vi "4-channel oscilloscope v1.01.vi"() -> ()   [LabVIEW 2014]
doc: "This example shows how to configure multiple channels and acquire waveforms from multiple channels."
uses:
  <vilib>/Analysis/Matrix/Datatypes/RealMatrix.ctl
  <instrlib>/Tektronix TDS 200 1000 2000 Series/Tektronix TDS 200 1000 2000 Series.lvlib
  <vilib>/Analysis/Matrix/NI_Matrix.lvlib
panel:
  out "Real Matrix":T1
  in  "Channel 4 (3: Channel 4)":u16(ring) items=["Channel 1", "Channel 2", "Channel 3", "Channel 4", "Math", "Reference A", "Reference B", "Reference C", "Reference D"]
  in  "Probe Attenuation 4 (0.1)":dbl=10.0
  in  "Vertical Coupling 4 (1: DC)":u16(ring)=1 items=["AC", "DC", "Ground"]
  in  "Channel 3 (2: Channel 3)":u16(ring) items=["Channel 1", "Channel 2", "Channel 3", "Channel 4", "Math", "Reference A", "Reference B", "Reference C", "Reference D"]
  in  "Probe Attenuation 3 (0.1)":dbl=10.0
  in  "Vertical Coupling 3 (1: DC)":u16(ring)=1 items=["AC", "DC", "Ground"]
  in  "Channel 2 (1: Channel 2)":u16(ring)=1 items=["Channel 1", "Channel 2", "Channel 3", "Channel 4", "Math", "Reference A", "Reference B", "Reference C", "Reference D"]
  in  "Channel 1 (0: Channel 1)":u16(ring) items=["Channel 1", "Channel 2", "Channel 3", "Channel 4", "Math", "Reference A", "Reference B", "Reference C", "Reference D"]
  in  "Serial Configuration":T2={"Baud Rate"=9600, "Parity"=0, "Stop Bits"=10, "Flow Control"=2} {"Flow Control" items=["None", "XON/XOFF", "RTS/CTS", "XON/XOFF & RTS/CTS", "DTR/DSR", "XON/XOFF & DTR/DSR"]; "Stop Bits" items=["1.0"=10, "1.5"=15, "2.0"=20]; "Parity" items=["None", "Odd", "Even", "Mark", "Space"]; "Baud Rate" items=["300"=300, "600"=600, "1200"=1200, "2400"=2400, "4800"=4800, "9600"=9600, "19200"=19200]}
  in  "Probe Attenuation 2 (0.1)":dbl=1.0
  in  "Vertical Coupling 2 (1: DC)":u16(ring)=1 items=["AC", "DC", "Ground"]
  in  "Probe Attenuation 1 (0.1)":dbl=10.0
  in  "Vertical Coupling 1 (1: DC)":u16(ring)=1 items=["AC", "DC", "Ground"]
  in  "Timeout (10000 ms)":u32=10000
  out "Waveform Data":waveform(dbl)[](graph)
  in  "VISA resource name":refnum<visa-resource-name>
  # "2015 NanoBEEs"
  # "Channel 3"
  # "Channel 1"
  # "Channel 2"
  # "Channel 4"
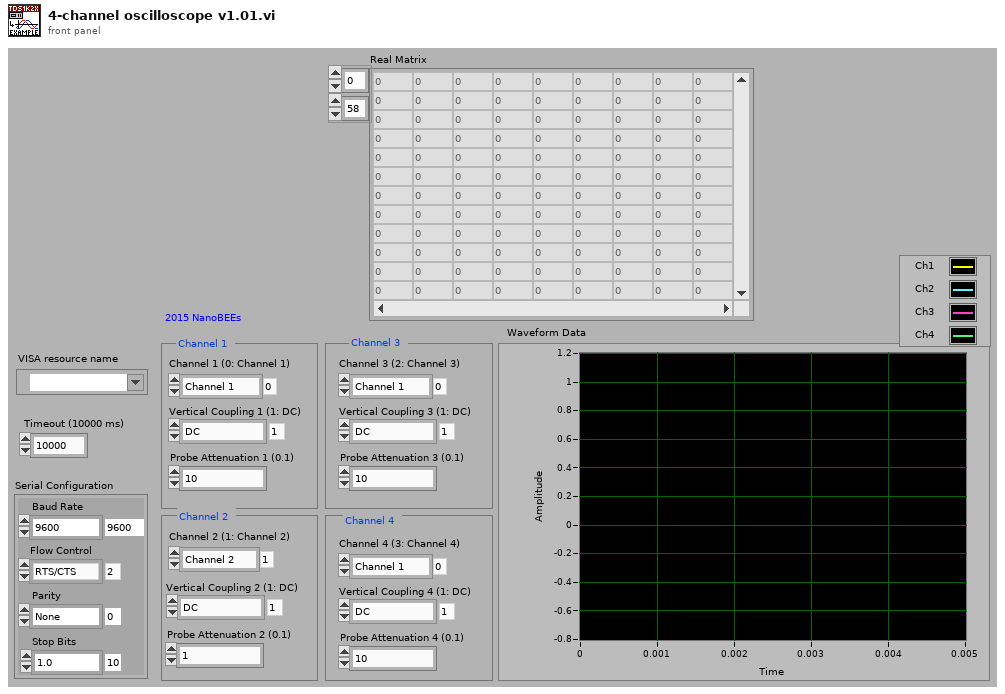
[diagram p1: front panel]
types:
  T1 = typedef "NI_Matrix.lvlib/RealMatrix.ctl" = dbl[][]
  T2 = cluster{"Baud Rate":u32, "Parity":u16, "Stop Bits":u16, "Flow Control":u16}
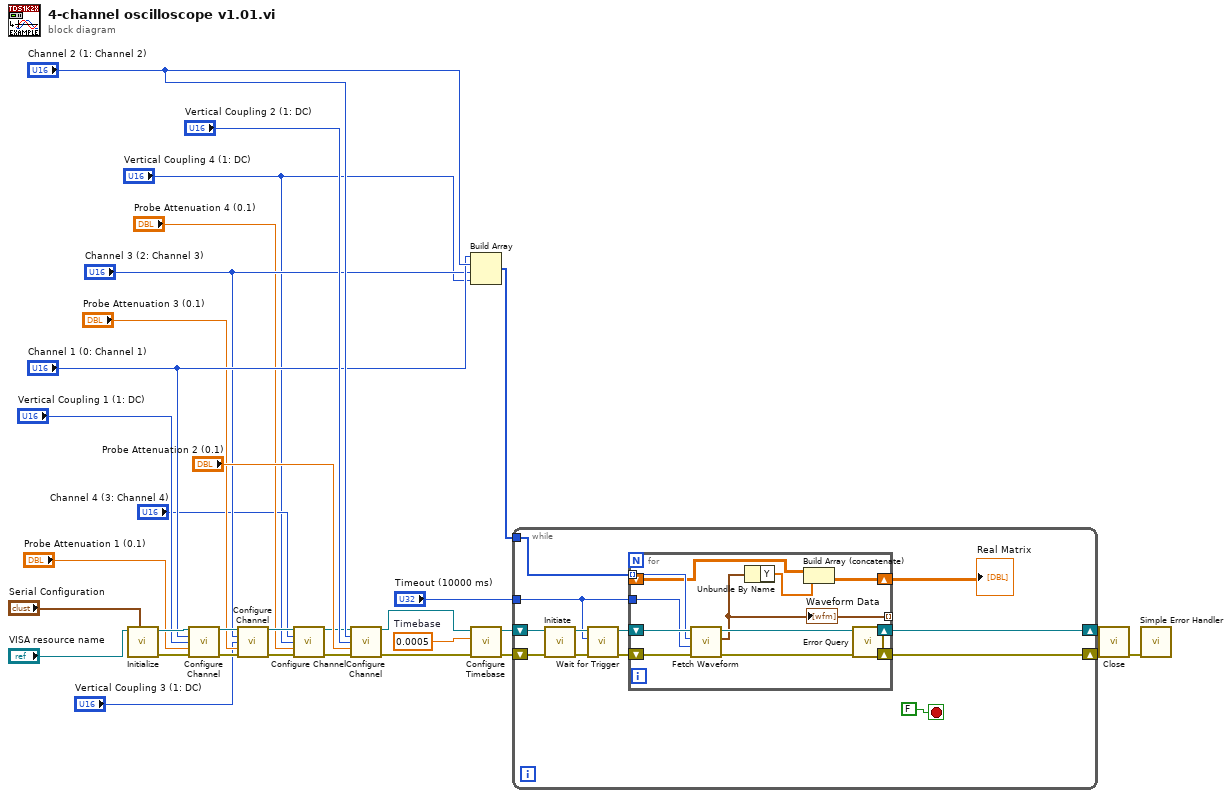
[diagram p0: block diagram]
diagram:
  w18 = 0.0005  # Timebase
  n1 = call <instrlib>:"Initialize.vi"("Serial Configuration"="Serial Configuration", "VISA resource name"="VISA resource name") -> ("error out"=w27:errorcluster, "VISA resource name out"=w28:refnum<visa-resource-name>)  [unwired: 3 in, 5 out]
  n2 = call <instrlib>:"Configure Channel.vi"("VISA resource name"=w28, "Channel (0: Channel 1)"="Channel 1 (0: Channel 1)", "Vertical Coupling (1: DC)"="Vertical Coupling 1 (1: DC)", "Probe Attenuation (10: 10X)"="Probe Attenuation 1 (0.1)", "error in (no error)"=w27) -> ("VISA resource name out"=w12:refnum<visa-resource-name>, "error out"=w9:errorcluster)  [unwired: 4 in, 5 out]
  n3 = call <instrlib>:"Configure Channel.vi"("VISA resource name"=w12, "Channel (0: Channel 1)"="Channel 3 (2: Channel 3)", "Vertical Coupling (1: DC)"="Vertical Coupling 3 (1: DC)", "Probe Attenuation (10: 10X)"="Probe Attenuation 3 (0.1)", "error in (no error)"=w9) -> ("VISA resource name out"=w11:refnum<visa-resource-name>, "error out"=w8:errorcluster)  [unwired: 4 in, 5 out]
  n4 = call <instrlib>:"Configure Channel.vi"("VISA resource name"=w11, "Channel (0: Channel 1)"="Channel 4 (3: Channel 4)", "Vertical Coupling (1: DC)"="Vertical Coupling 4 (1: DC)", "Probe Attenuation (10: 10X)"="Probe Attenuation 4 (0.1)", "error in (no error)"=w8) -> ("VISA resource name out"=w10:refnum<visa-resource-name>, "error out"=w7:errorcluster)  [unwired: 4 in, 5 out]
  n5 = call <instrlib>:"Configure Channel.vi"("VISA resource name"=w10, "Channel (0: Channel 1)"="Channel 2 (1: Channel 2)", "Vertical Coupling (1: DC)"="Vertical Coupling 2 (1: DC)", "Probe Attenuation (10: 10X)"="Probe Attenuation 2 (0.1)", "error in (no error)"=w7) -> ("VISA resource name out"=w26:refnum<visa-resource-name>, "error out"=w25:errorcluster)  [unwired: 4 in, 5 out]
  n6 = Build Array("Channel 1 (0: Channel 1)", "Channel 2 (1: Channel 2)", "Channel 3 (2: Channel 3)", "Vertical Coupling 4 (1: DC)") -> (w16:u16[])
  n7 = call <instrlib>:"Configure Timebase.vi"("error in (no error)"=w25, "Timebase (0.0005 s)"=w18, "VISA resource name"=w26) -> ("error out"=w23:errorcluster, "VISA resource name out"=w24:refnum<visa-resource-name>)  [unwired: 1 in, 6 out]
  n8 = while {
    tunnel: w16 -> [w40]
    tunnel: "Timeout (10000 ms)" -> [w39]
    shift-right: [w36] -> w30
    shift-left: w24 -> [w38]
    shift-right: [w35] -> w29
    shift-left: w23 -> [w37]
    stop <- FALSE stop-if-true
    n9 = call <instrlib>:"Initiate.vi"("error in (no error)"=w37, "VISA resource name"=w38) -> ("error out"=w41:errorcluster, "VISA resource name out"=w44:refnum<visa-resource-name>)  [unwired: 8 out]
    n10 = call <instrlib>:"Wait for Trigger.vi"("error in (no error)"=w41, "Timeout (10000 ms)"=w39, "VISA resource name"=w44) -> ("error out"=w42:errorcluster, "VISA resource name out"=w43:refnum<visa-resource-name>)  [unwired: 7 out]
    n11 = for {
      shift-right: [w56] -> w45
      shift-left: w42 -> [w54]
      tunnel: w40 -> [w52] mode=indexing
      tunnel: [w51] -> w34 mode=indexing
      tunnel: w39 -> [w53]
      shift-right: [w57] -> w46
      shift-left: w43 -> [w55]
      shift-right: [w49] -> w33
      shift-left: _ -> [w48]
      n12 = call <instrlib>:"Fetch Waveform.vi"("error in (no error)"=w54, "Timeout (10000 ms)"=w53, "Source (0: Channel 1)"=w52, "VISA resource name"=w55) -> ("error out"=w56:errorcluster, "Waveform Data"=w51:waveform(dbl), "VISA resource name out"=w57:refnum<visa-resource-name>)  [unwired: 2 in, 3 out]
      n13 = Unbundle By Name(w51) -> ("Y"=w50:dbl[])
      n14 = Build Array (concatenate)(w48, w50) -> (w49:T1)
    }
    "Waveform Data" <- w34
    "Real Matrix" <- w33
    n15 = call <instrlib>:"Error Query.vi"("error in (no error)"=w45, "VISA resource name"=w46) -> ("error out"=w35:errorcluster, "VISA resource name out"=w36:refnum<visa-resource-name>)  [unwired: 8 out]
  }
  n16 = call <instrlib>:"Close.vi"("error in (no error)"=w29, "VISA resource name"=w30) -> ("error out"=w31:errorcluster)  [unwired: 9 out]
  n17 = call <vilib>:"Simple Error Handler.vi"("error in (no error)"=w31) -> ()  [unwired: 1 in, 8 out]
